vi "oax_gsColor Map.vi"() -> ()   [LabVIEW 2017]
doc: "This is Order Analysis Toolkit demo VI."
uses:
  <vilib>/addons/Sound and Vibration/Order Analysis/Tach Process/SoundVib_TachProcess.lvlib
  <vilib>/Waveform/WDTOps.llb/WDT Waveform Duration DBL.vi
  <vilib>/addons/Sound and Vibration/Order Analysis/Resample Order Tracking/SoundVib_OrderTracking.lvlib
  <vilib>/addons/_XControls/Colormap/SVX Colormap.xctl
panel:
  out "Colormap":T1(xcontrol)
  in  "windows info":cluster{"window type":u32, "window length":i32}={"window type"=62, "window length"=2048} {"window length" min=2; "window type" items=["None"=0, "Hanning"=1, "Hamming"=2, "Blackman-Harris"=3, "Exact Blackman"=4, "Blackman"=5, "Flat Top"=6, "4 Term B-Harris"=7, "7 Term B-Harris"=8, "Low Sidelobe"=9, "Gaussian"=62]}
  in  "dB on? (T)":bool=TRUE
  in  "Select Data":i32(listbox)
  in  "STOP":bool
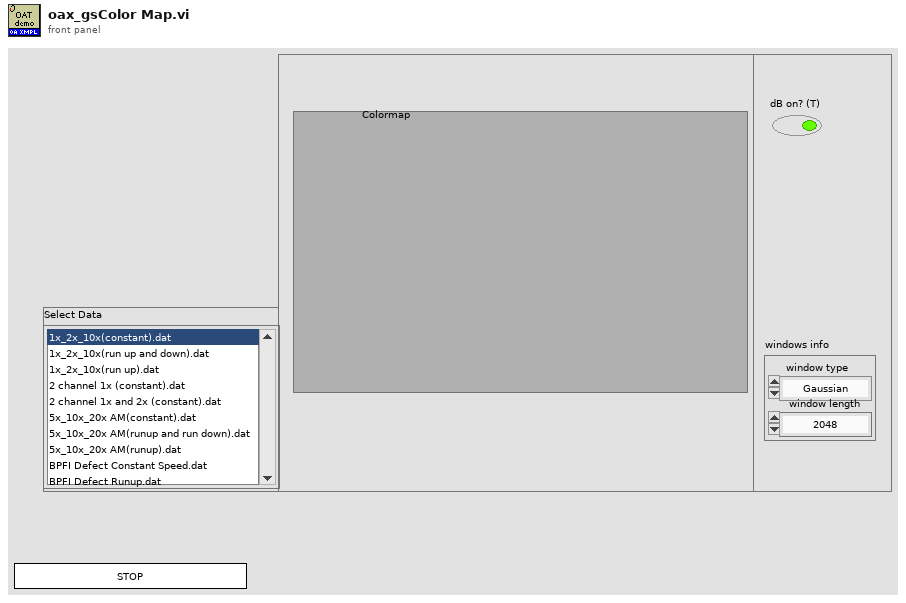
[diagram p1: front panel]
types:
  T1 = cluster{"spectral map":dbl[][], "X scale":cluster{"offset":dbl, "multiplier":dbl}, "Y scale":cluster{"offset":dbl, "multiplier":dbl}, "attribute":variant}
  T2 = enum16{"Frequency-Time", "Time-Frequency", "Order-Time", "Time-Order"}
  T3 = typedef "SoundVib_TachProcess.lvlib/speed profile.ctl" = cluster{"time [s]":dbl[], "speed [RPM]":dbl[]}
  T4 = cluster{"value":dbl[][], "x scale":cluster{"offset":dbl, "multiplier":dbl}, "y scale":cluster{"offset":dbl, "multiplier":dbl}, "attribute":variant}
  T5 = cluster{"x-axis unit label":string, "y-axis unit label":string, "z-axis unit label":string}
  T6 = cluster{"pulse / rev":i32, "threshold (auto)":dbl, "slope (Rising)":u16}
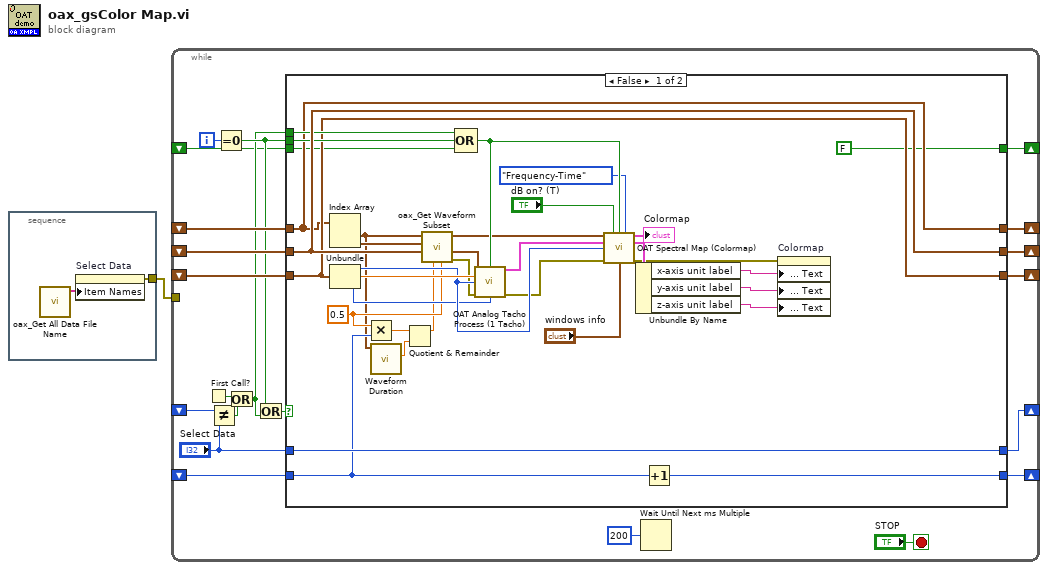
[diagram p0: block diagram]
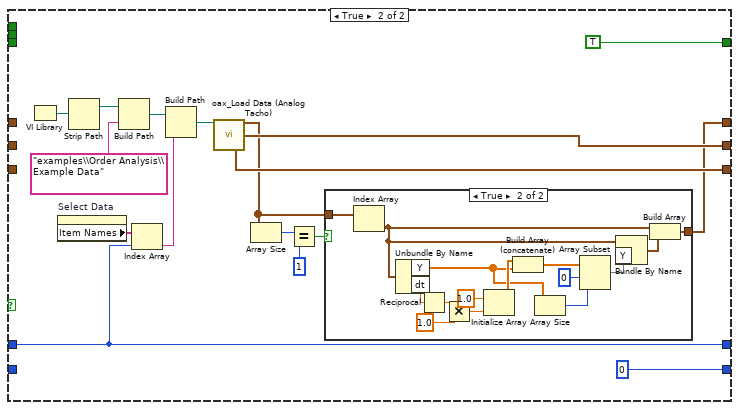
[diagram p2: hidden frame]
diagram:
  n1 = stacked-sequence {
    tunnel: [w2] -> w1
    frame #0 {
      n2 = call <vilib>:"oax_Get All Data File Name.vi"() -> ("file names"=w3:string[])  [unwired: 10 in, 1 out]
      n3 = property on="Select Data" class="LstBox (strict)"("Item Names"=w3) -> (error out=w2:errorcluster)  [unwired: 2 in, 1 out]
    }
  }
  n4 = while {
    shift-right: [w20] -> _
    shift-left: _ -> [w21]
    shift-right: [w18] -> _
    shift-left: _ -> [w24]
    shift-right: [w17] -> _
    shift-left: _ -> [w22]
    shift-right: [w16] -> _
    shift-left: _ -> [w15]
    tunnel: w1 -> [_]
    shift-right: [w6] -> _
    shift-left: _ -> [w7]
    shift-right: [w5] -> _
    shift-left: _ -> [w4]
    i -> [w14]
    stop <- "STOP" stop-if-true
    n5 = First Call?() -> (First Call?: T/F=w10:bool)
    n6 = Not Equal?(x=w21, y="Select Data") -> (x != y?=w9:bool)
    n7 = Equal To 0?(x=w14) -> (x = 0?=w13:bool)
    n8 = Or(x=w10, y=w9) -> (x .or. y?=w8:bool)
    n9 = Or(x=w13, y=w8) -> (x .or. y?=w12:bool)
    n10 = case shown="False" w12 {
      tunnel: w24 -> [w38 _]
      tunnel: w22 -> [w56 _]
      tunnel: [w57 w74] -> w20
      tunnel: "Select Data" -> [w57 w74]
      tunnel: [w38 w59] -> w18
      tunnel: [w56 w72] -> w17
      tunnel: [w49 w71] -> w16
      tunnel: w15 -> [w49 _]
      tunnel: w8 -> [w54 _]
      tunnel: w13 -> [w53 _]
      tunnel: w7 -> [w43 _]
      tunnel: [w45 0] -> w6
      tunnel: [FALSE TRUE] -> w5
      tunnel: w4 -> [w37 _]
      frame False {
        w44 = 0.5 ("y")
        n11 = Index Array(array=w38) -> (element #1=w42:waveform(dbl), element #2=w50:waveform(dbl))  [unwired: 2 in]
        n12 = Unbundle(w49) -> ("pulse / rev"=w47:i32, "threshold (auto)"=w48:dbl, "slope (Rising)"=w46:u16)
        n13 = Multiply(x=w44, y=w43) -> (x*y=w40:dbl)
        n14 = call-poly <vilib>:"Waveform Duration.vi"("waveform in"=w42) -> ("duration"=w41:dbl)  [unwired: 8 in, 2 out]
        n15 = Quotient & Remainder(x=w40, y=w41) -> (x-y*floor(x/y)=w39:dbl)  [unwired: 1 out]
        n16 = call <vilib>:"oax_Get Waveform Subset.vi"("duration"=w44, "start index"=w39, "Tach Signal"=w56, "Vibration Signal Y"=w50, "Vibration Signal X"=w42) -> ("error out"=w31:errorcluster, "Tach Signal out"=w55:waveform(dbl), "Vibration Signal X out"=w51:waveform(dbl))  [unwired: 3 in, 1 out]
        n17 = Compound Arithmetic op=OR(w54, w53, w37) -> (w52:bool)
        n18 = call <vilib>:"OAT Analog Tacho Process (1 Tacho).vi"("analog tacho signal"=w55, "reset? (F)"=w52, "threshold (auto)"=w48, "pulse/revolution (1)"=w47, "error in (no error)"=w31, "slope (Rising)"=w46) -> ("speed profile"=w58:T3, "error out"=w30:errorcluster)  [unwired: 5 in, 3 out]
        n19 = call <vilib>:"OAT Spectral Map (Colormap).vi"("scaled signal [EU]"=w51, "dB on? (T)"="dB on? (T)", "reset? (F)"=w52, "plot type"=T2."Frequency-Time", "speed profile"=w58, "pulse/revolution (1)"=w47, "error in (no error)"=w30, "windows info"="windows info") -> ("colormap"=→"Colormap":T4, "colormap unit labels"=w32:T5, "error out"=w29:errorcluster)  [unwired: 3 in, 2 out]
        n20 = Unbundle By Name(w32) -> ("x-axis unit label"=w26:string, "y-axis unit label"=w27:string, "z-axis unit label"=w28:string)
        n21 = Increment(x=w43) -> (x+1=w45:i32)
        n22 = property on="Colormap"(error in=w29, "X Scale: Name Label: Text"=w26, "Y Scale: Name Label: Text"=w27, "Z Scale: Name Label: Text"=w28) -> ()  [unwired: 1 in, 2 out]
      }
      frame True {
        n23 = VI Library() -> (path=w67:path)
        n24 = property on="Select Data" class="LstBox (strict)"() -> ("Item Names"=w75:string[])  [unwired: 2 in, 2 out]
        n25 = Strip Path(path=w67) -> (stripped path=w66:path)  [unwired: 1 out]
        n26 = Build Path(base path=w66, name or relative path="examples\\Order Analysis\\Example Data") -> (appended path=w70:path)
        n27 = Index Array(array=w75, index=w74) -> (element=w69:string)
        n28 = Build Path(base path=w70, name or relative path=w69) -> (appended path=w68:path)
        n29 = call <vilib>:"oax_Load Data (Analog Tacho).vi"("Data Path In"=w68) -> ("vibration data"=w60:waveform(dbl)[], "analog tacho signal"=w72:waveform(dbl), "tacho info"=w71:T6)  [unwired: 8 in, 4 out]
        n30 = Array Size(array=w60) -> (size(s)=w63:i32)
        n31 = Equal?(x=w63, y=1) -> (x = y?=w61:bool)
        n32 = case shown="True" w61 {
          tunnel: w60 -> [w76 w91]
          tunnel: [w76 w90] -> w59
          frame False {
          }
          frame True {
            n33 = Index Array(array=w91) -> (element=w89:waveform(dbl))  [unwired: 1 in]
            n34 = Unbundle By Name(w89) -> ("Y"=w78:dbl[], "dt"=w87:dbl)
            n35 = Reciprocal(x=w87) -> (1/x=w86:dbl)
            n36 = Multiply(x=w86, y=1.0) -> (x*y=w84:dbl)
            n37 = Initialize Array(1.0 ("element"), w84) -> (w80:dbl[])
            n38 = Build Array (concatenate)(w80, w78) -> (w82:dbl[])
            n39 = Array Size(array=w78) -> (size(s)=w79:i32)
            n40 = Array Subset(array=w82, index=0, length=w79) -> (w77:dbl[])
            n41 = Bundle By Name(cluster=w89, "Y"=w77) -> (w88:waveform(dbl))
            n42 = Build Array(w89, w88) -> (w90:waveform(dbl)[])
          }
        }
      }
    }
    n43 = Wait Until Next ms Multiple(millisecond multiple=u32 200) -> ()  [unwired: 1 out]
  }
